vi "InitFichierTlog.vi"(4 "error in (no error)":errorcluster, 5 "JourDernSauv":i32, 6 "Répertoire initial":path=path "C:/Données/Run003", 7 "Entête":string) -> (0 "error out":errorcluster, 1 "Jour Actuel":i32, 2 "CheminSauv":path=path "C:/Données/Run003" caption="Fichier de Sauvegarde")   [LabVIEW 2010]
doc: "Ce VI ouvre ou crée le fichier de sauvegarde à partir de la date du jour ou du nom spécifié et il y sauvegarde l'entête des colonnes de données"
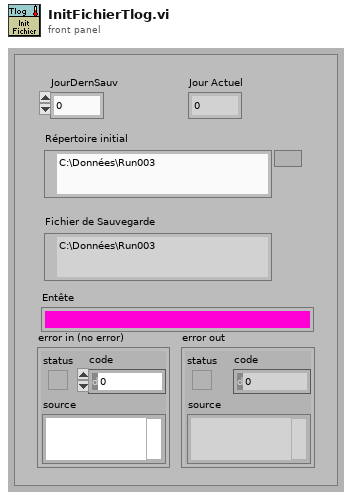
[diagram p1: front panel]
types:
  T1 = enum16{"open", "open or create", "create or replace", "create", "open (read only)"}
  T2 = cluster{"second":i32, "minute":i32, "hour":i32, "day of month":i32, "month":i32, "year":i32, "day of week":i32, "day of year":i32, "is DST":i32}
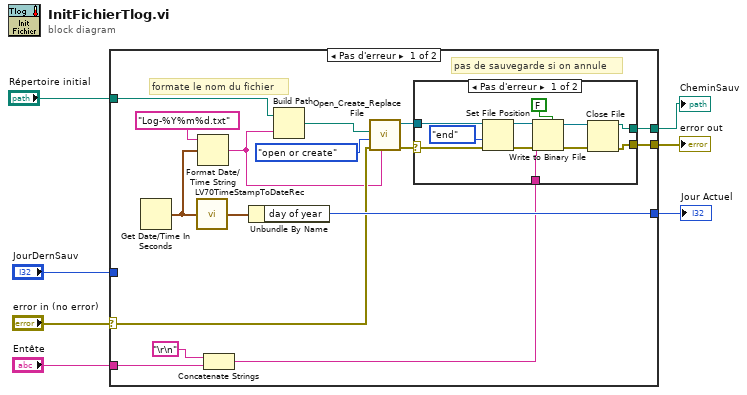
[diagram p0: block diagram]
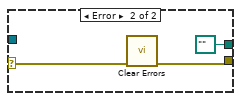
[diagram p2: hidden frame]
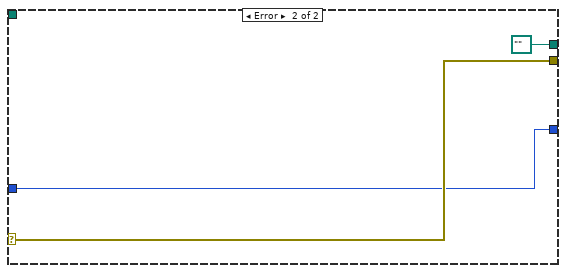
[diagram p3: hidden frame]
diagram:
  n1 = case shown="Pas d'erreur" "error in (no error)" {
    selector: "error in (no error)" -> [w11 w40]
    tunnel: [w22 w39] -> w7
    tunnel: "Répertoire initial" -> [w18 _]
    tunnel: [w16 w40] -> w5
    tunnel: [w15 path "" ("path")] -> w4
    tunnel: "Entête" -> [w14 _]
    tunnel: "JourDernSauv" -> [_ w39]
    frame No Error {
      # "formate le nom du fichier"
      # "pas de sauvegarde si on annule"
      n2 = Get Date/Time In Seconds() -> (seconds since 1Jan1904=w20:timestamp)
      n3 = call <vilib>:"LV70TimeStampToDateRec.vi"("time stamp"=w20) -> ("date time rec"=w23:T2)
      n4 = Format Date/Time String(time format string (%c)="Log-%Y%m%d.txt", seconds (now)=w20) -> (date/time string=w9:string)  [unwired: 1 in]
      n5 = Concatenate Strings("\r\n", w14) -> (w13:string)
      n6 = Unbundle By Name(w23) -> ("day of year"=w22:i32)
      n7 = Build Path(base path=w18, name or relative path=w9) -> (appended path=w10:path)
      n8 = call <vilib>:"Open_Create_Replace File.vi"("default name"=w9, "error in (no error)"=w11, "function (open:0)"=T1."open or create", "start path  (Not A Path)"=w10) -> ("error out"=w8:errorcluster, "refnum"=w17:refnum<file>)  [unwired: 4 in, 2 out]
      n9 = case shown="Pas d'erreur" w8 {
        selector: w8 -> [w27 w37]
        tunnel: w17 -> [w31 _]
        tunnel: [w30 w36] -> w16
        tunnel: [w29 path "" ("path")] -> w15
        tunnel: w13 -> [w28 _]
        frame No Error {
          n10 = Set File Position(refnum=w31, from (0:start)=enum16{"start", "end", "current"}."end" ("pos mode (0:2)"), error in=w27) -> (refnum out=w26:refnum<file>, error out=w25:errorcluster)  [unwired: 1 in]
          n11 = Write to Binary File(file (use dialog)=w26, data=w28, error in=w25, 5:FALSE ("ajouter une taille de tableau ou de chaîne ? (V)")) -> (refnum out=w32:refnum<file>, error out=w34:errorcluster)  [unwired: 2 in, 1 out]
          n12 = Close File(refnum=w32, error in=w34) -> (path=w29:path, error out=w30:errorcluster)
        }
        frame Error {
          n13 = call <vilib>:"Clear Errors.vi"("error in (no error)"=w37) -> ("error out"=w36:errorcluster)  [unwired: 6 in]
        }
      }
    }
    frame Error {
    }
  }
  "error out" <- w5
  "Jour Actuel" <- w7
  "CheminSauv" <- w4
